vi "Write name.vi"(8 "error in (no error)":errorcluster, 10 "name":string, 11 "MagFieldTable in":refnum<class "MagFieldTable.lvclass">) -> (0 "error out":errorcluster, 3 "MagFieldTable out":refnum<class "MagFieldTable.lvclass">)   [LabVIEW 2018, in "MagFieldTable.lvclass"]
doc: "writes the name of the MFT (same as section in ini-file)"
uses:
  MagFieldTable.lvclass
  MagFieldTable.lvclass/MagFieldTable.ctl
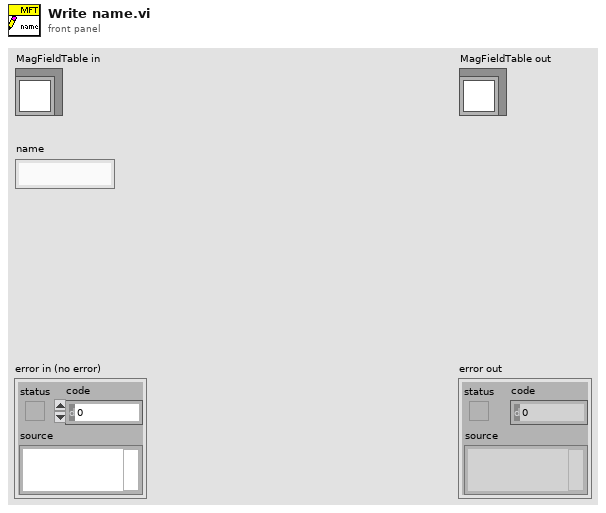
[diagram p1: front panel]
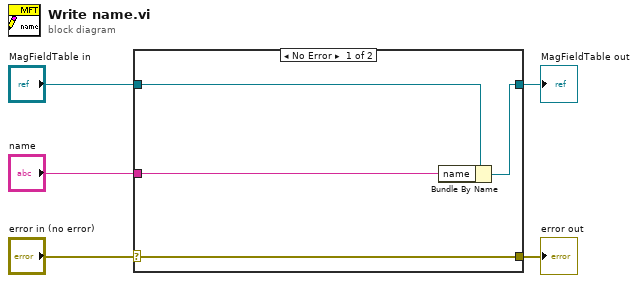
[diagram p0: block diagram]
diagram:
  n1 = case shown="No Error" "error in (no error)" {
    selector: "error in (no error)" -> [w9 w10]
    tunnel: [w9 w10] -> w4
    tunnel: [w7 w11] -> w2
    tunnel: "MagFieldTable in" -> [w8 w11]
    tunnel: "name" -> [w6 _]
    frame No Error {
      n2 = Bundle By Name(cluster=w8, "name"=w6) -> (w7:refnum<class "MagFieldTable.lvclass">)
    }
    frame Error {
    }
  }
  "error out" <- w4
  "MagFieldTable out" <- w2
